vi "Add.vi"(8 "error in (no error)":errorcluster, 11 "LV MDI in":refnum<class "LV MDI.lvclass">) -> (0 "error out":errorcluster, 3 "LV MDI out":refnum<class "LV MDI.lvclass">)   [LabVIEW 2016, in "LV MDI.lvclass"]
doc: "Add VI to the container and display it within the container."
uses:
  LV MDI.lvclass
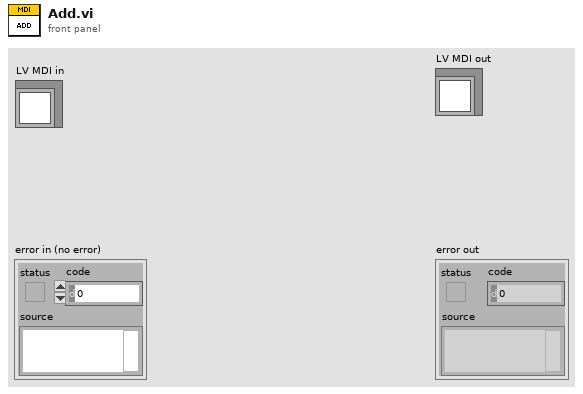
[diagram p1: front panel]
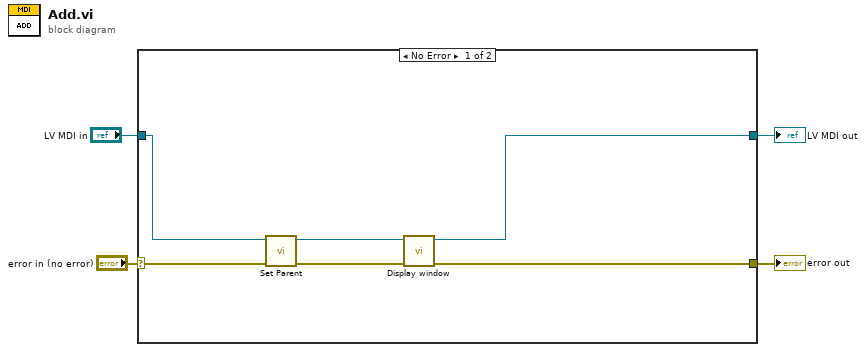
[diagram p0: block diagram]
diagram:
  n1 = case shown="No Error" "error in (no error)" {
    selector: "error in (no error)" -> [w10 w12]
    tunnel: [w7 w12] -> w3
    tunnel: [w5 w11] -> w1
    tunnel: "LV MDI in" -> [w8 w11]
    frame No Error {
      n2 = call "Set Parent.vi"("error in (no error)"=w10, "LV MDI in"=w8) -> ("error out"=w9:errorcluster, "LV MDI out"=w6:refnum<class "LV MDI.lvclass">)  [unwired: 8 in]
      n3 = call "Display window.vi"("error in (no error)"=w9, "LV MDI in"=w6) -> ("error out"=w7:errorcluster, "LV MDI out"=w5:refnum<class "LV MDI.lvclass">)  [unwired: 8 in]
    }
    frame Error {
    }
  }
  "error out" <- w3
  "LV MDI out" <- w1
